vi "LRC checker.vi"(11 "Data In":u8[](array[numeric]) format="%.0x") -> (2 "Valid?":bool, 3 "Function Data Out":u8[](array[numeric]) format="%.0x")   [LabVIEW 2021, in "ASCII Data Unit.lvclass"]
doc: "this is where the magic happens."
uses:
  ASCII Data Unit.lvclass
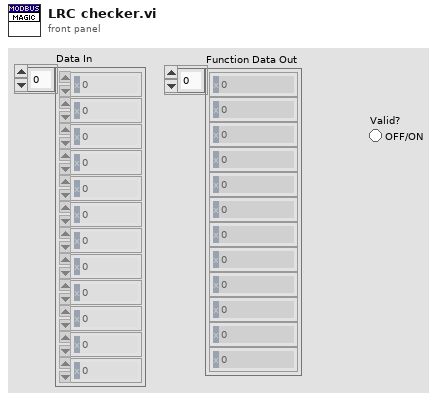
[diagram p1: front panel]
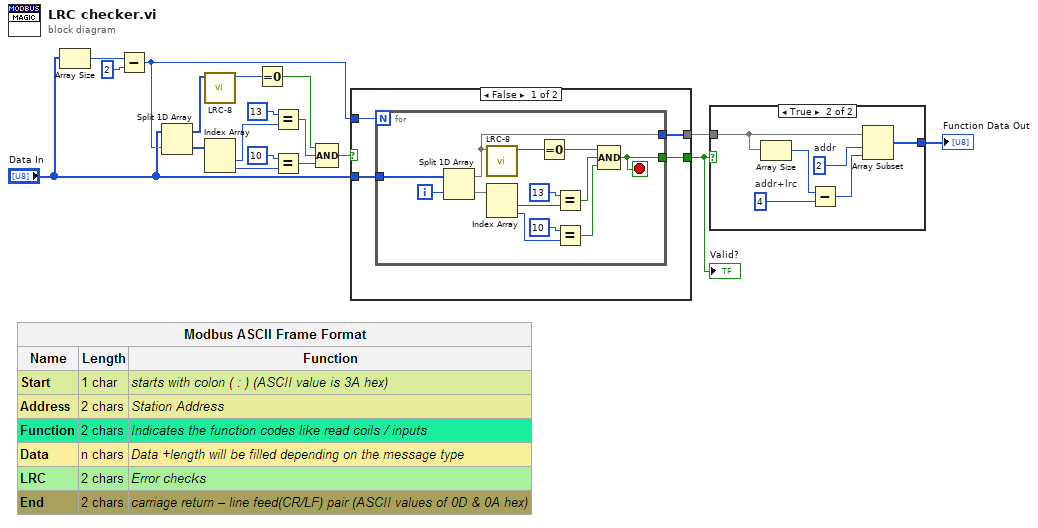
[diagram p0: block diagram]
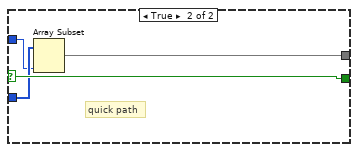
[diagram p2: hidden frame]
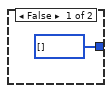
[diagram p3: hidden frame]
diagram:
  n1 = Array Size(array="Data In") -> (size(s)=w9:i32)
  n2 = Subtract(x=w9, y=2 ("x")) -> (x-y=w5:i32)
  n3 = Split 1D Array(array="Data In", index=w5) -> (first subarray=w2:u8[], second subarray=w3:u8[])
  n4 = call "LRC-8.vi"("data"=w2) -> ("LRC-8"=w4:u8)  [unwired: 10 in]
  n5 = Index Array(array=w3) -> (element #1=w12:u8, element #2=w15:u8)  [unwired: 2 in]
  n6 = Equal To 0?(x=w4) -> (x = 0?=w1:bool)
  n7 = Equal?(x=u8 13, y=w12) -> (x = y?=w10:bool)
  n8 = Equal?(x=u8 10, y=w15) -> (x = y?=w11:bool)
  n9 = Compound Arithmetic op=AND(w1, w10, w11) -> (w7:bool)
  n10 = case shown="False" w7 {
    selector: w7 -> [_ w39]
    tunnel: [w22 w36] -> w18
    tunnel: [w21 w39] -> w17
    tunnel: "Data In" -> [w20 w38]
    tunnel: w5 -> [w19 w37]
    frame False {
      n11 = for {
        N: w19 -> [_]
        tunnel: w20 -> [w31]
        tunnel: [w24] -> w22
        tunnel: [w23] -> w21
        i -> [w30]
        stop <- w23 stop-if-true
        n12 = Split 1D Array(array=w31, index=w30) -> (first subarray=w24:u8[], second subarray=w29:u8[])
        n13 = call "LRC-8.vi"("data"=w24) -> ("LRC-8"=w28:u8)  [unwired: 10 in]
        n14 = Index Array(array=w29) -> (element #1=w35:u8, element #2=w32:u8)  [unwired: 2 in]
        n15 = Equal To 0?(x=w28) -> (x = 0?=w27:bool)
        n16 = Equal?(x=u8 13, y=w35) -> (x = y?=w26:bool)
        n17 = Equal?(x=u8 10, y=w32) -> (x = y?=w25:bool)
        n18 = Compound Arithmetic op=AND(w27, w26, w25) -> (w23:bool)
      }
    }
    frame True {
      # "quick path"
      n19 = Array Subset(array=w38, length=w37) -> (w36:u8[])  [unwired: 1 in]
    }
  }
  "Valid?" <- w17
  n20 = case shown="True" w17 {
    tunnel: w18 -> [_ w44]
    tunnel: [u8[] [] w41] -> w16
    frame False {
    }
    frame True {
      w43 = 2  # addr
      w45 = 4  # addr+lrc
      n21 = Array Size(array=w44) -> (size(s)=w46:i32)
      n22 = Subtract(x=w46, y=w45) -> (x-y=w42:i32)
      n23 = Array Subset(array=w44, index=w43, length=w42) -> (w41:u8[])
    }
  }
  "Function Data Out" <- w16
